vi "Destroy.vi"(8 "error in (no error)":errorcluster, 11 "Font in":refnum<class "Sprite Font.lvclass">) -> (0 "error out":errorcluster)   [LabVIEW 2021, in "Sprite Font.lvclass"]
uses:
  Sprite Font.lvclass
  Sprite Font.lvclass/Sprite Font.ctl
  Resource Manager/Resource Manager.lvclass
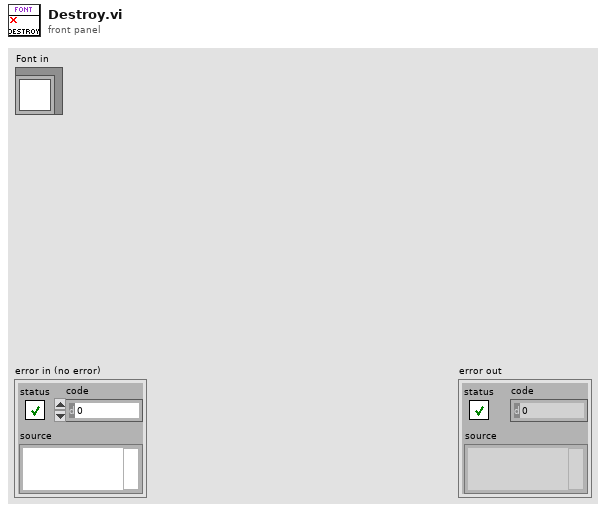
[diagram p1: front panel]
types:
  T1 = typedef "Sprite Font.lvclass/Character.ctl" = cluster{"Texture Name":string, "Size":refnum<class "Vector 2D.lvclass">}
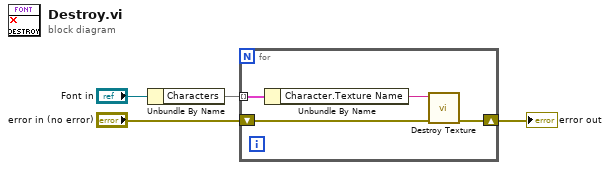
[diagram p0: block diagram]
diagram:
  n1 = Unbundle By Name("Font in") -> ("Characters"=w4:map{string, T1})
  n2 = for {
    shift-right: [w7] -> w2
    shift-left: "error in (no error)" -> [w8]
    tunnel: w4 -> [w6] mode=indexing
    n3 = Unbundle By Name(w6) -> ("Character.Texture Name"=w5:string)
    n4 = call "Destroy Texture.vi"("error in (no error)"=w8, "Texture Name"=w5) -> ("error out"=w7:errorcluster)  [unwired: 9 in]
  }
  "error out" <- w2
